vi "Bung_Tue_Gi.vi"(11 "Raw_PPG":dbl[](array[numeric])) -> (3 "reference":dbl[](array[numeric]))   [LabVIEW 2014]
panel:
  out "size":dbl
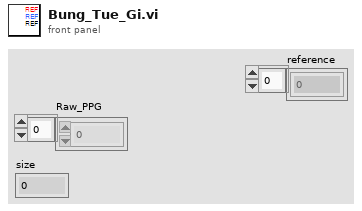
[diagram p1: front panel]
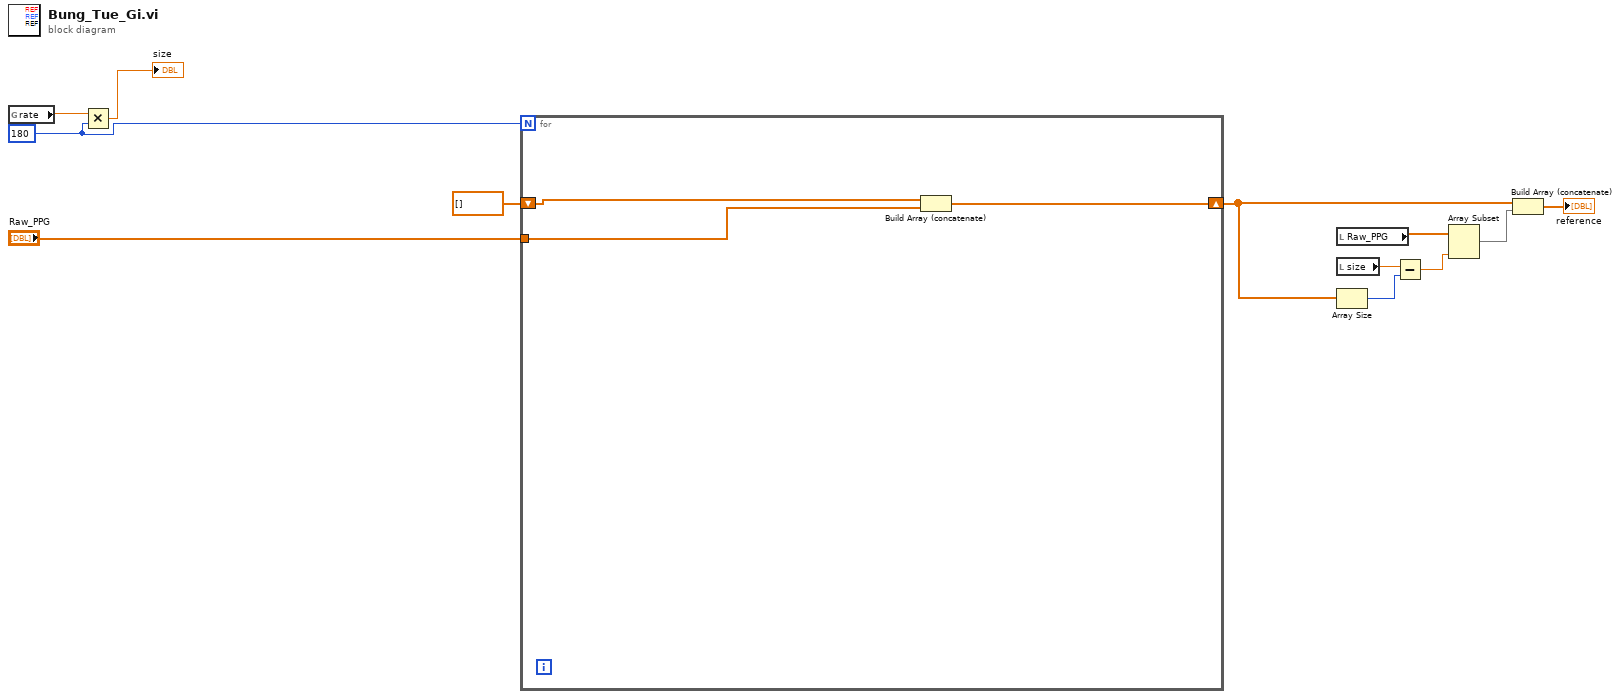
[diagram p0: block diagram]
diagram:
  w3 = 180
  n1 = global read "Control_Panel.vi" "rate"() -> (w12:dbl)
  n2 = Multiply(x=w12, y=w3) -> (x*y=→"size":dbl)
  n3 = for {
    N: w3 -> [_]
    tunnel: "Raw_PPG" -> [w15]
    shift-right: [w14] -> w6
    shift-left: dbl[] [] -> [w13]
    n4 = Build Array (concatenate)(w13, w15) -> (w14:dbl[])
  }
  n5 = local read "Raw_PPG"() -> (w7:dbl[])
  n6 = local read "size"() -> (w10:dbl)
  n7 = Array Size(array=w6) -> (size(s)=w9:i32)
  n8 = Subtract(x=w10, y=w9) -> (x-y=w8:dbl)
  n9 = Array Subset(array=w7, length=w8) -> (w5:dbl[])  [unwired: 1 in]
  n10 = Build Array (concatenate)(w6, w5) -> (→"reference":dbl[])
